vi "Write All Chnl Param2CnfgFile.vi"(8 "error in (no error)":errorcluster, 11 "BME_DG_System in":refnum<class "BME_DG_System.lvclass">) -> (0 "error out":errorcluster, 3 "BME_DG_System out":refnum<class "BME_DG_System.lvclass">)   [LabVIEW 2009, in "POLARIS BME DG.lvlib" / "BME_DG_System.lvclass"]
uses:
  BME_DG_System.lvclass
  BME_DG_System.lvclass/BME_DG_System.ctl
  BME_DG_Base/BME_DG_Base.lvclass
  BME_DG_Chnl/BME_DG_Chnl.lvclass
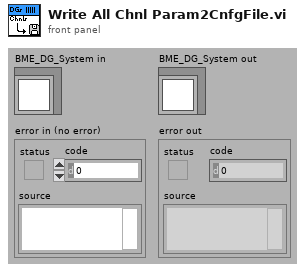
[diagram p1: front panel]
types:
  T1 = typedef "POLARIS BME DG.lvlib/DetectDG.ctl" = cluster{"DG_Number":i32, "DG_Product":i32, "Product Name":string, "Bus_Number":i32, "Slot_Number":i32, "Master":bool}
  T2 = typedef "POLARIS BME DG.lvlib/System DG Selection.ctl" = cluster{"Selected System DGs":T1[], "Name":string}
  T3 = typedef "POLARIS BME DG.lvlib/Card Config.ctl" = cluster{"Logical Name":string, "Base Settings":T4, "SG08_Settings":T6, "Channel Names":string[], "Advanced Settings":T7}
  T4 = typedef "POLARIS BME DG.lvlib/BME_DG_TriggerSettings.ctl" = cluster{"Clock Source":T5, " clock modulo":u32, "TriggerEnabled?":bool, "trigger modulo ":i32, "InputTerminated?":bool, "Inhibit(µs)":dbl, "TriggerLevel":dbl, "PresetValue":i32, "InternalTrigger?":bool, "InternalArm?":bool, "SWTrigger?":bool, "RisingEdge?":bool, "StopOnPreset?":bool, "ResetWhenDone?":bool, "Gate Divider":i32, "PositiveGate?":bool}
  T5 = typedef "POLARIS BME DG.lvlib/ClockSource.ctl" = i32
  T6 = typedef "POLARIS BME DG.lvlib/SG08_Settings.ctl" = cluster{"Gate Terminate":bool, "Gate Level":dbl, "Gate Delay (µs)":dbl, "StepBackTime (µs)":dbl, "Burst Counter":u32, "Trigger Divider":u32, "Trigger Multiplier":u32}
  T7 = typedef "POLARIS BME DG.lvlib/BME_DG_V2TriggerSettings.ctl" = cluster{"Trigger on MS Bus":T8, "Force Trigger (µs)":dbl, "Gate Type":bool, "Synchronize Gate":bool}
  T8 = typedef "POLARIS BME DG.lvlib/MSBusSignals.ctl" = u32
  T9 = typedef "POLARIS BME DG.lvlib/Chnl Settings Complete.ctl" = cluster{"Channel Name":string, "ChnParameter":T10, "DelayFormula":string, "OutputModulo":i32, "Go and Done Signal":T11, "G08_Chnl_Settings":T13}
  T10 = typedef "POLARIS BME DG.lvlib/ChnlSettings.ctl" = cluster{" Delay (µs)":dbl, "On?":bool, "PositiveVoltage?":bool, "50OhmTerminated? ":bool, "25OhmOutput?":bool}
  T11 = typedef "POLARIS BME DG.lvlib/Go_Done_Chnl_Settings.ctl" = cluster{"Go Signal":T12, "Done Signal":u32}
  T12 = typedef "POLARIS BME DG.lvlib/GoSignalBits.ctl" = u32
  T13 = typedef "POLARIS BME DG.lvlib/SG08_Chnl_Settings.ctl" = cluster{"Pulse Width (µs)":dbl, "Output Offset":u32, "Disconnect (E,F)":bool, "Onto MsBus (E,F)":bool, "Input Positive (E,F)":bool}
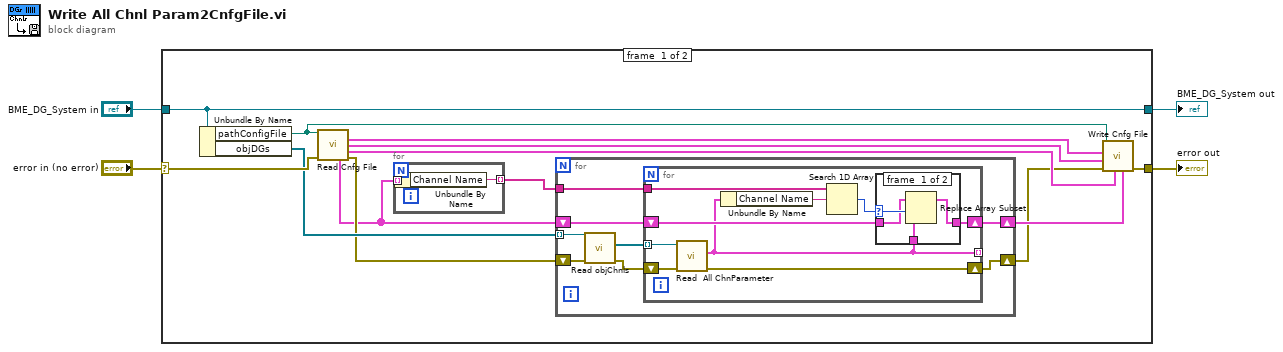
[diagram p0: block diagram]
diagram:
  n1 = case shown="No Error" "error in (no error)" {
    selector: "error in (no error)" -> [w12 w43]
    tunnel: [w11 w43] -> w3
    tunnel: [w17 w42] -> w1
    tunnel: "BME_DG_System in" -> [w17 w42]
    frame #0 {
      n2 = Unbundle By Name(w17) -> ("pathConfigFile"=w13:path, "objDGs"=w10:refnum<class "BME_DG_Base.lvclass">[])
      n3 = call "Read Cnfg File.vi"("Config File"=w13, "error in (no error)"=w12) -> ("InstalledDGs"=w16:T1[], "DGSystems"=w15:T2[], "Cards"=w14:T3[], "Chnls"=w6:T9[], "error out"=w8:errorcluster)  [unwired: 8 in, 1 out]
      n4 = for {
        tunnel: w6 -> [w19] mode=indexing
        tunnel: [w18] -> w5 mode=indexing
        n5 = Unbundle By Name(w19) -> ("Channel Name"=w18:string)
      }
      n6 = for {
        tunnel: w10 -> [w27] mode=indexing
        shift-right: [w20] -> w9
        shift-left: w6 -> [w21]
        shift-right: [w23] -> w7
        shift-left: w8 -> [w25]
        tunnel: w5 -> [w22]
        n7 = call-dynamic "Read objChnls.vi"("error in (no error)"=w25, "BME_DG_Base in"=w27) -> ("error out"=w24:errorcluster, "objChnls"=w26:refnum<class "BME_DG_Chnl.lvclass">[])  [unwired: 6 in, 2 out]
        n8 = for {
          tunnel: w26 -> [w36] mode=indexing
          tunnel: [w28] -> _ mode=indexing
          shift-right: [w34] -> w23
          shift-left: w24 -> [w35]
          tunnel: w22 -> [w33]
          shift-right: [w29] -> w20
          shift-left: w21 -> [w30]
          n9 = call-dynamic "Read  All ChnParameter.vi"("error in (no error)"=w35, "BME_DG_Chnl in"=w36) -> ("error out"=w34:errorcluster, "ChnlParam"=w28:T9)  [unwired: 7 in, 1 out]
          n10 = Unbundle By Name(w28) -> ("Channel Name"=w32:string)
          n11 = Search 1D Array(1D array=w33, element=w32) -> (index of element=w31:i32)  [unwired: 1 in]
          n12 = case shown="0, Default" w31 {
            selector: w31 -> [w40 _]
            tunnel: w30 -> [w39 w41]
            tunnel: [w37 w41] -> w29
            tunnel: w28 -> [w38 _]
            frame #0 {
              n13 = Replace Array Subset(array=w39, new element=w38, index=w40) -> (w37:T9[])
            }
            frame #1 {
            }
          }
        }
      }
      n14 = call "Write Cnfg File.vi"("Chnls"=w9, "Cards"=w14, "error in"=w7, "DGSystems"=w15, "InstalledDGs"=w16, "pathConfigFile"=w13) -> ("error out"=w11:errorcluster)  [unwired: 4 in, 1 out]
    }
    frame #1 {
    }
  }
  "error out" <- w3
  "BME_DG_System out" <- w1
